vi "Open Excel.vi"(2 "error in (no error)":errorcluster caption="错误输入（无错误）", 3 "Visible Boolean":bool=TRUE caption="可见布尔") -> (0 "error out":errorcluster caption="错误输出", 1 "Excel._Application":refnum<k7>)   [LabVIEW 2014]
doc: "本VI将通过创建Excel.Application对象的自动化句柄以打开Excel。根据可见输入控件，该VI会将“可见”属性设置为真或假。"
panel:
  in  "Excel._Application":refnum<k7>
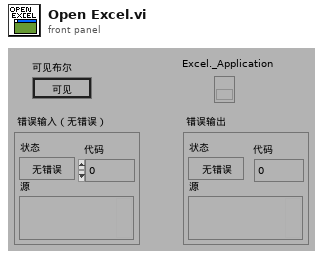
[diagram p1: front panel]
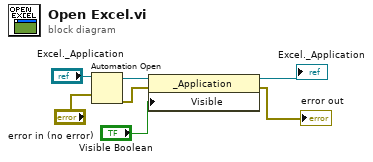
[diagram p0: block diagram]
diagram:
  n1 = Automation Open(error in (no error)="error in (no error)", Automation Refnum="Excel._Application") -> (Automation Refnum=w4:refnum<k7>, error out=w3:errorcluster)  [unwired: 2 out]
  n2 = property class="_Application"(reference=w4, error in=w3, "Visible"="Visible Boolean") -> (reference out=→"Excel._Application":refnum<k7>, error out=→"error out":errorcluster)
